vi "CenterRectInBnds.vi"(8 "错误输入":errorcluster, 10 "bounds":T1 caption="边界", 11 "rect":T1 caption="矩形") -> (0 "错误输出":errorcluster, 3 "centered rect":T1 caption="居中矩形")   [LabVIEW 2012, in "Picture Box Tools.lvlib" / "Rect Tools.lvlib"]
uses:
  Rect Tools.lvlib
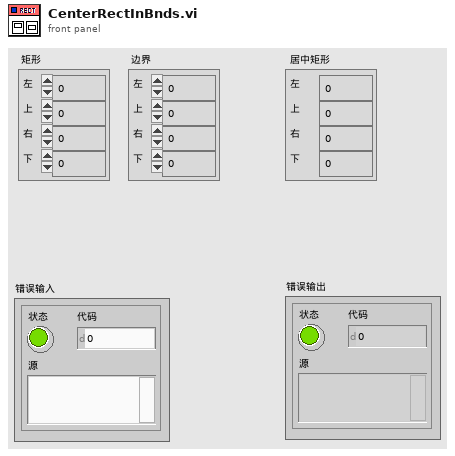
[diagram p1: front panel]
types:
  T1 = cluster{"left":i16, "top":i16, "right":i16, "bottom":i16}
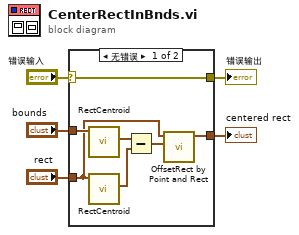
[diagram p0: block diagram]
diagram:
  n1 = case shown="无错误" "错误输入" {
    selector: "错误输入" -> [w9 w14]
    tunnel: [w9 w14] -> w4
    tunnel: "bounds" -> [w8 _]
    tunnel: "rect" -> [w7 w13]
    tunnel: [w6 w13] -> w1
    frame No Error {
      n2 = call "RectCentroid.vi"("Rect In"=w8) -> ("point"=w12:cluster{"x":i16, "y":i16})  [unwired: 8 in, 2 out]
      n3 = call "RectCentroid.vi"("Rect In"=w7) -> ("point"=w11:cluster{"x":i16, "y":i16})  [unwired: 8 in, 2 out]
      n4 = Subtract(x=w12, y=w11) -> (x-y=w10:cluster{"x":i16, "y":i16})
      n5 = call "OffsetRect by Point and Rect.vi"("point"=w10, "rect"=w7) -> ("offset rect"=w6:T1)  [unwired: 8 in, 1 out]
    }
    frame Error {
    }
  }
  "错误输出" <- w4
  "centered rect" <- w1
